vi "Animate Charm.vi"(8 "error in (no error)":errorcluster, 9 "Smooth?":bool=TRUE, 10 "Direction":T1, 11 "MainController in":refnum<class "MainController.lvclass">) -> (0 "error out":errorcluster, 3 "MainController out":refnum<class "MainController.lvclass">)   [LabVIEW 2012, in "Win8uiFramework.lvlib" / "MainController.lvclass"]
uses:
  MainController.lvclass
  Visibility Direction.ctl
  ViewableActor.lvclass/ViewableActor.ctl
  MainController.lvclass/MainController.ctl
  Read UI VI Ref.vi
  Read Charm Splitter.vi
  Win8uiFramework.lvlib
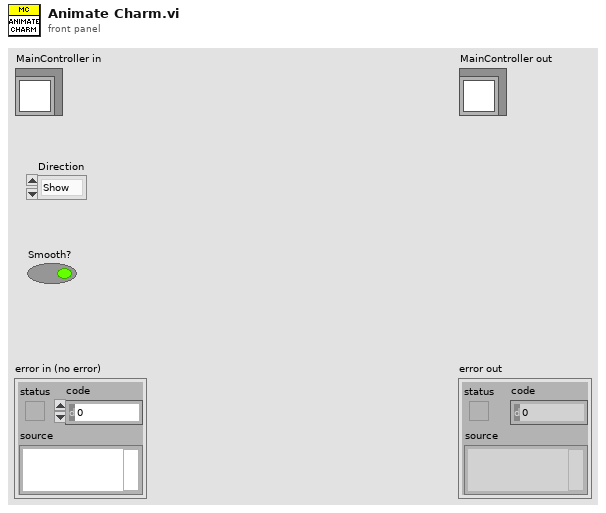
[diagram p1: front panel]
types:
  T1 = typedef "Win8uiFramework.lvlib/Visibility Direction.ctl" = enum16{"Show", "Hide"}
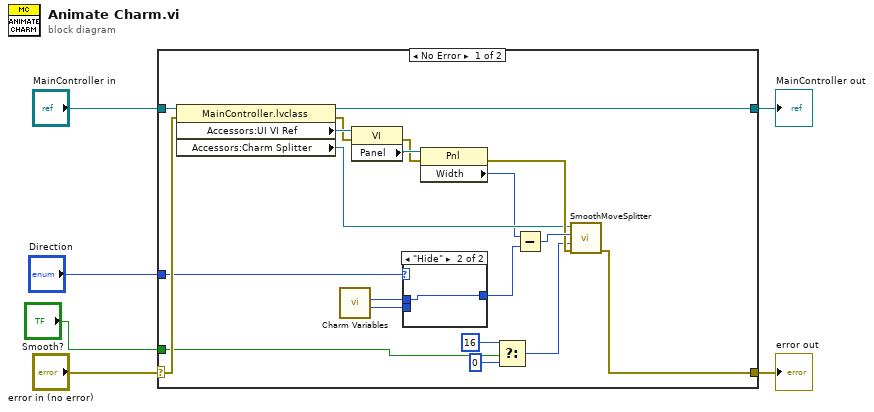
[diagram p0: block diagram]
diagram:
  n1 = case shown="No Error" "error in (no error)" {
    selector: "error in (no error)" -> [w18 w30]
    tunnel: [w17 w30] -> w5
    tunnel: [w25 w29] -> w3
    tunnel: "MainController in" -> [w26 w29]
    tunnel: "Direction" -> [w15 _]
    tunnel: "Smooth?" -> [w10 _]
    frame No Error {
      n2 = property class="MainController.lvclass"(reference=w26, error in=w18) -> (reference out=w25:refnum<class "MainController.lvclass">, error out=w21:errorcluster, "Accessors:UI VI Ref"=w23:refnum<vi>, "Accessors:Charm Splitter"=w12:refnum<vi>)
      n3 = call "Charm Variables.vi"() -> ("Charm Width"=w13:i32, "Charm Peek Width"=w14:u32)  [unwired: 10 in]
      n4 = property class="VI"(reference=w23, error in=w21) -> (error out=w20:errorcluster, "Panel"=w24:refnum<vi>)  [unwired: 1 out]
      n5 = case shown="\"Hide\"" w15 {
        tunnel: w13 -> [w27 _]
        tunnel: [w27 w28] -> w16
        tunnel: w14 -> [_ w28]
        frame "Show", Default {
        }
        frame "Hide" {
        }
      }
      n6 = property class="Pnl"(reference=w24, error in=w20) -> (error out=w19:errorcluster, "Width"=w11:u32)  [unwired: 1 out]
      n7 = Select(t=16 ("Steps (16)"), s=w10, f=0) -> (s? t:f=w7:i32)
      n8 = Subtract(x=w11, y=w16) -> (x-y=w22:u32)
      n9 = call "SmoothMoveSplitter.vi"("error in (no error)"=w19, "Steps (16)"=w7, "Position"=w22, "Splitter in"=w12) -> ("error out"=w17:errorcluster)  [unwired: 7 in]
    }
    frame Error {
    }
  }
  "error out" <- w5
  "MainController out" <- w3
